vi "Destroy.vi"(0 "reference in":refnum<class "DemoSubSubClass1.lvclass">, 5 "error in (no error)":errorcluster) -> (14 "reference out":refnum<class "DemoSubSubClass1.lvclass">, 19 "error out":errorcluster)   [LabVIEW 2020, in "DemoSubSubClass1.lvclass"]
uses:
  DemoSubSubClass1.lvclass
  C:/ProjectGSharpDevelopment_2020-3/gsharp/VIPM/Files/vi.lib/addons/_AddQ/G#Object/G#Object.lvclass
  DemoSubClass1_class/DemoSubClass1.lvclass
  vi.lib/addons/_AddQ/G#Object/G#Object.lvclass
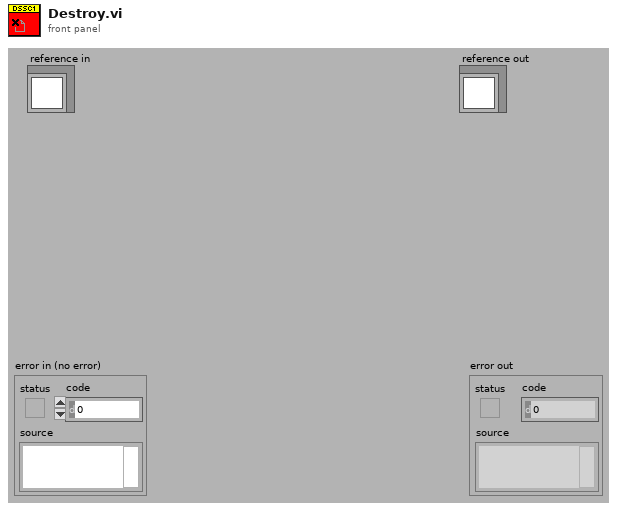
[diagram p1: front panel]
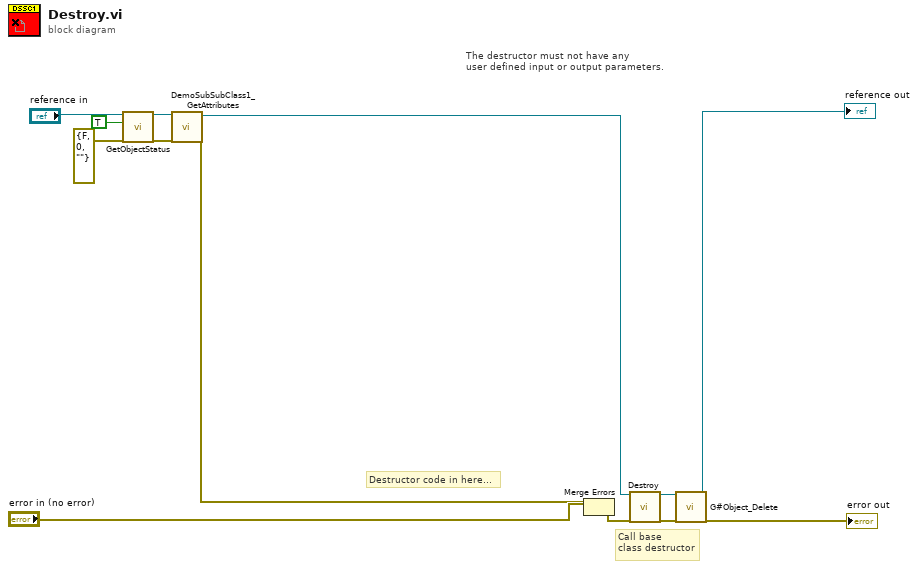
[diagram p0: block diagram]
diagram:
  # "Destructor code in here..."
  # "The destructor must not have any\nuser defined input or output parameters."
  # "Call base\nclass destructor"
  n1 = call-dynamic "GetObjectStatus.vi"("reference in"="reference in", "simple info (F)"=TRUE ("Simple Info"), "error in (no error)"=errorcluster {"status"=FALSE, "code"=0, "source"=""}) -> ("reference out"=w5:refnum<class "DemoSubSubClass1.lvclass">, "error out"=w3:errorcluster)  [unwired: 5 in, 10 out]
  n2 = call "DemoSubSubClass1_GetAttributes.vi"("reference in"=w5, "error in (no error)"=w3) -> ("reference out"=w9:refnum<class "DemoSubSubClass1.lvclass">, "error out"=w6:errorcluster)  [unwired: 1 in, 15 out]
  n3 = Merge Errors("error in (no error)", w6) -> (w12:errorcluster)
  n4 = call-parent "Destroy.vi"("reference in"=w9, "error in (no error)"=w12) -> ("reference out"=w8:refnum<class "DemoSubSubClass1.lvclass">, "error out"=w11:errorcluster)  [unwired: 16 out]
  n5 = call "G#Object_Delete.vi"("reference in"=w8, "error in (no error)"=w11) -> ("reference out"=→"reference out":refnum<class "DemoSubSubClass1.lvclass">, "error out"=→"error out":errorcluster)  [unwired: 16 in]
